vi "DOWN.vi"() -> (3 "DOWN":T1)   [LabVIEW 2023, in "d17.lvlib"]
uses:
  d17.lvlib
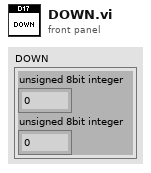
[diagram p1: front panel]
types:
  T1 = cluster{"unsigned 8bit integer":i16, "unsigned 8bit integer":i16}
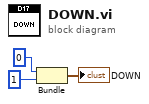
[diagram p0: block diagram]
diagram:
  n1 = Bundle("unsigned 8bit integer"=i16 0, "unsigned 8bit integer"=i16 1) -> (→"DOWN":T1)  [unwired: 1 in]
